vi "Create.vi"(9 "Alias":string, 10 "Actor":refnum<class "Actor.lvclass">, 11 "Process in":refnum<class "Process.lvclass">) -> (0 "error out":errorcluster, 3 "Process out":refnum<class "Process.lvclass">)   [LabVIEW 2021, in "Process.lvlib" / "Process.lvclass"]
uses:
  Process.lvclass
  AAM/AAM/Actor/Actor.lvclass
  Process.lvclass/Process.ctl
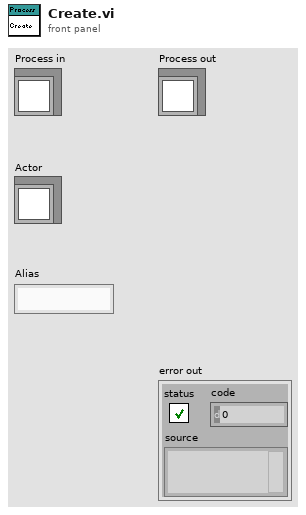
[diagram p1: front panel]
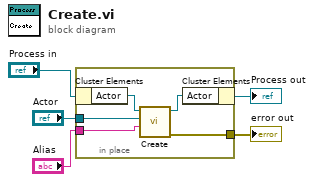
[diagram p0: block diagram]
diagram:
  n1 = in-place {
    in-place-border: "Actor" -> [w8]
    in-place-border: "Alias" -> [w7]
    in-place-border: [w6] -> w2
    n2 = in-place-cluster #1("Process in") -> ("Actor"=w10:refnum<class "Actor.lvclass">)
    n3 = call-dynamic "Create.vi"("Alias"=w7, "Actor"=w8, "Create in"=w10) -> ("error out"=w6:errorcluster, "Create out"=w9:refnum<class "Actor.lvclass">)  [unwired: 7 in]
    n4 = in-place-cluster #1("Actor"=w9) -> (→"Process out":refnum<class "Process.lvclass">)
  }
  "error out" <- w2
